vi "write new connection message.vi"(11 "connection":refnum<class "connection maintainer.lvclass">) -> (3 "element":refnum<class "communicator message.lvclass">)   [LabVIEW 2015, in "connection maintainer.lvclass"]
uses:
  connection maintainer.lvclass
  message/communicator message.lvclass
  message/communicator message.lvclass/communicator message.ctl
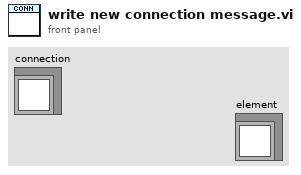
[diagram p1: front panel]
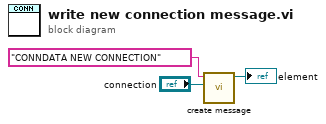
[diagram p0: block diagram]
diagram:
  n1 = call "create message.vi"("data"="connection", "ID"="CONNDATA NEW CONNECTION") -> ("message"=→"element":refnum<class "communicator message.lvclass">)  [unwired: 9 in]
